vi "DoInit.vi"(8 "error in (no error)":errorcluster, 11 "MainMenu in":refnum<class "MainMenu.lvclass">) -> (0 "error out":errorcluster, 3 "MainMenu out":refnum<class "MainMenu.lvclass">)   [LabVIEW 2019, in "RT_Game.lvlib" / "MainMenu.lvclass"]
uses:
  MainMenu.lvclass
  C:/Users/FreshBob/Dropbox/VIs/myRIO_GameConsole/RT/RT_Game/Menu/Menu.lvclass
  SnakeGame/SnakeGame.lvclass
  C:/Users/FreshBob/Dropbox/VIs/myRIO_GameConsole/RT/RT_Game/Game/Game.lvclass
  SnakeGame/SnakeGame.lvclass/SnakeGame.ctl
  Menu/Menu.lvclass/Menu.ctl
  MainMenu.lvclass/MainMenu.ctl
  SnakeGame/Write SinglePlayer.vi
  Menu/Write Entries.vi
  Menu/Menu.lvclass
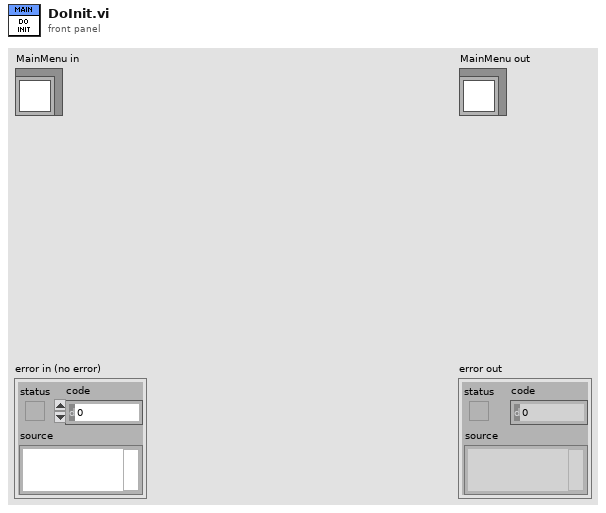
[diagram p1: front panel]
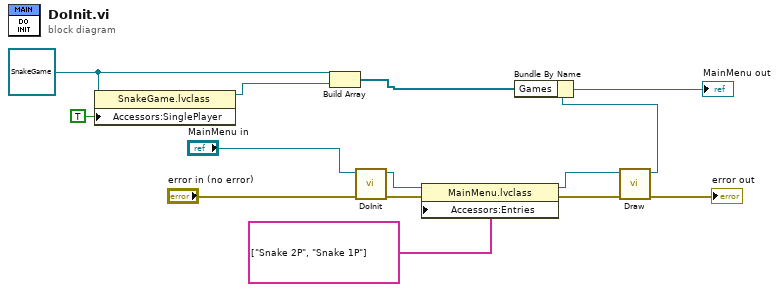
[diagram p0: block diagram]
diagram:
  w9 = refnum<class "SnakeGame.lvclass"> refnum ("RT_Game.lvlib:Snake.lvclass")
  n1 = property class="SnakeGame.lvclass"(reference=w9, "Accessors:SinglePlayer"=TRUE ("SinglePlayer")) -> (reference out=w8:refnum<class "SnakeGame.lvclass">)  [unwired: 1 in, 1 out]
  n2 = Build Array(w9, w8) -> (w7:refnum<class "SnakeGame.lvclass">[])
  n3 = call-parent "DoInit.vi"("error in (no error)"="error in (no error)", "Menu in"="MainMenu in") -> ("error out"=w14:errorcluster, "Menu out"=w5:refnum<class "MainMenu.lvclass">)  [unwired: 8 in]
  n4 = property class="MainMenu.lvclass"(reference=w5, error in=w14, "Accessors:Entries"=string[] ["Snake 2P", "Snake 1P"] ("Entries")) -> (reference out=w2:refnum<class "MainMenu.lvclass">, error out=w6:errorcluster)
  n5 = call "Draw.vi"("error in (no error)"=w6, "Menu in"=w2) -> ("error out"=→"error out":errorcluster, "Menu out"=w1:refnum<class "MainMenu.lvclass">)  [unwired: 8 in]
  n6 = Bundle By Name(cluster=w1, "Games"=w7) -> (→"MainMenu out":refnum<class "MainMenu.lvclass">)
